vi "Correlation_Display.vi"(5 "Inst names":string[](array[string])=["HW 1", "HW 2"], 6 "OK":bool) -> (2 "correlation array":i32[][](array[numeric]) min=0 max=8)   [LabVIEW 2010]
uses:
  Globals/Meas_global.vi
panel:
  in  "number of correlation pairs":i32=1
  in  "correlation choices":i32[][](array[ring])=[[0, 1], [0, 0], [0, 0]] items=["LDA (U)", "LDA (W)", "HW (HW) Sync", "RV (WT) Sync", "HW (HW)", "RV (WT)"]
  # "1st Pair"
  # "2nd Pair"
  # "3rd Pair"
  # "4th Pair"
  # "5th Pair"
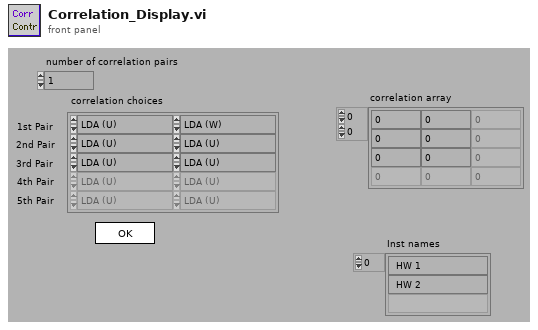
[diagram p1: front panel]
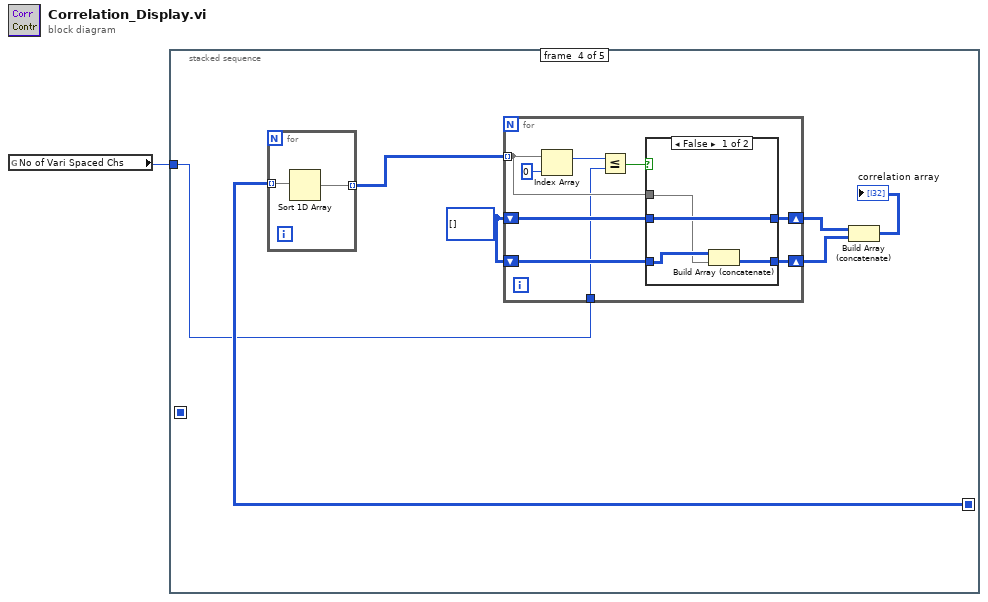
[diagram p0: block diagram]
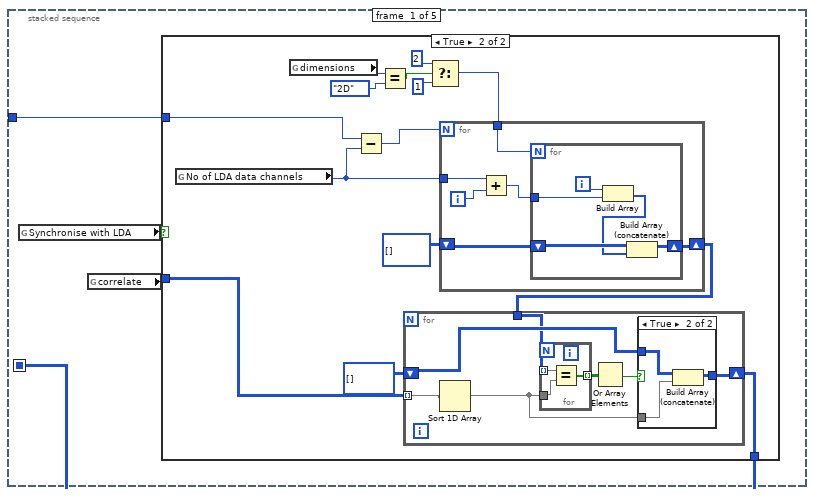
[diagram p2: hidden frame]
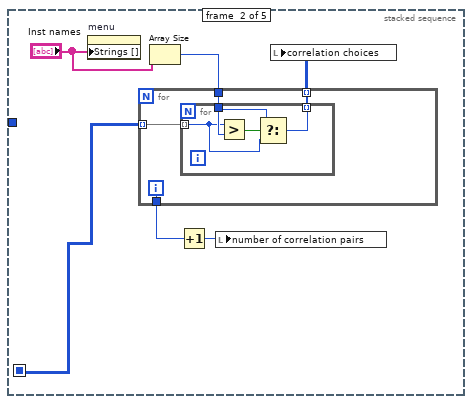
[diagram p5: hidden frame]
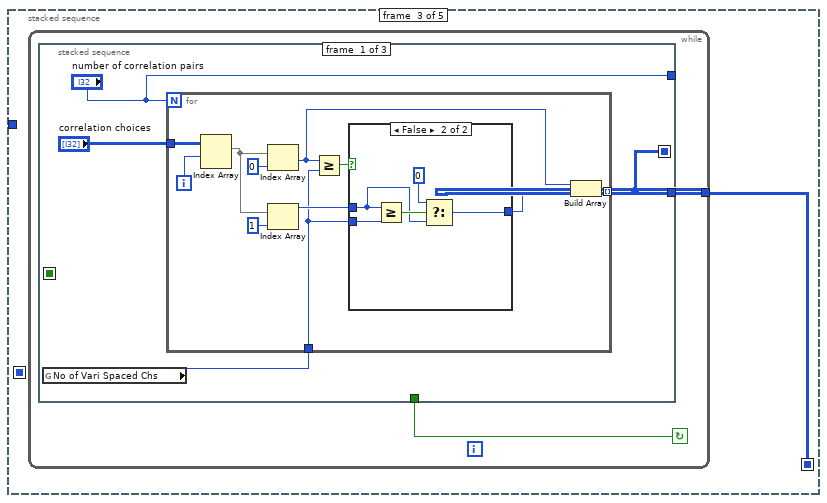
[diagram p6: hidden frame]
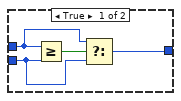
[diagram p7: hidden frame]
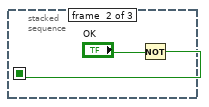
[diagram p8: hidden frame]
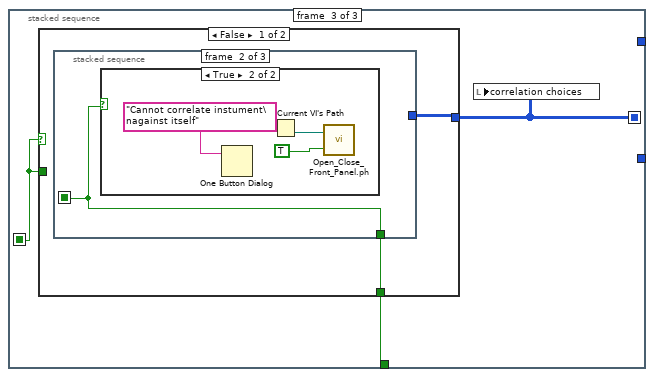
[diagram p9: hidden frame]
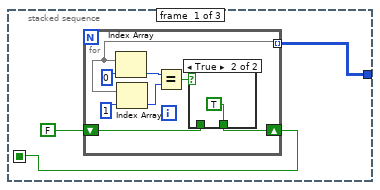
[diagram p10: hidden frame]
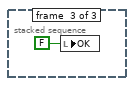
[diagram p13: hidden frame]
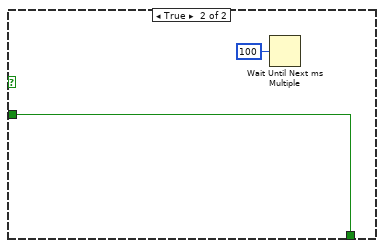
[diagram p14: hidden frame]
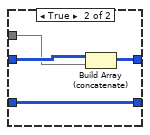
[diagram p15: hidden frame]
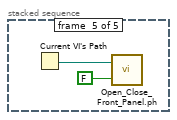
[diagram p16: hidden frame]
diagram:
  n1 = global read "Meas_global.vi" "No of Vari Spaced Chs"() -> (w1:i32)
  n2 = stacked-sequence {
    seq-local: [_ _ w60 _ _] -> [_ _ _ w120 _]
    seq-local: [w3 _ _ _ _] -> [_ w48 _ _ _]
    tunnel: w1 -> [w2 _ _ w117 _]
    frame #0 {
      n3 = global read "Meas_global.vi" "Synchronise with LDA"() -> (w5:bool)
      n4 = global read "Meas_global.vi" "correlate"() -> (w4:i32[][])
      n5 = case shown="True" w5 {
        tunnel: w4 -> [w6 w12]
        tunnel: [w6 w11] -> w3
        tunnel: w2 -> [_ w9]
        frame False {
        }
        frame True {
          n6 = global read "Meas_global.vi" "No of LDA data channels"() -> (w19:i32)
          n7 = global read "Meas_global.vi" "dimensions"() -> (w18:enum16{"1D", "2D"})
          n8 = Subtract(x=w9, y=w19) -> (x-y=w20:i32)
          n9 = Equal?(x=w18, y=enum16{"1D", "2D"}."2D" ("dimensions")) -> (x = y?=w16:bool)
          n10 = Select(t=2, s=w16, f=1) -> (s? t:f=w13:i32)
          n11 = for {
            N: w20 -> [_]
            tunnel: w19 -> [w40]
            tunnel: w13 -> [w38]
            shift-right: [w36] -> w7
            shift-left: i32[][] [] -> [w35]
            i -> [w39]
            n12 = Add(x=w40, y=w39) -> (x+y=w37:i32)
            n13 = for {
              N: w38 -> [_]
              tunnel: w37 -> [w44]
              shift-right: [w42] -> w36
              shift-left: w35 -> [w43]
              i -> [w45]
              n14 = Build Array(w45, w44) -> (w41:i32[])
              n15 = Build Array (concatenate)(w43, w41) -> (w42:i32[][])
            }
          }
          n16 = for {
            shift-right: [w25] -> w11
            shift-left: i32[][] [] -> [w22]
            tunnel: w12 -> [w24] mode=indexing
            tunnel: w7 -> [w21]
            n17 = Sort 1D Array(array=w24) -> (sorted array=w23:i32[])
            n18 = for {
              tunnel: w23 -> [w34]
              tunnel: w21 -> [w32] mode=indexing
              tunnel: [w33] -> w27 mode=indexing
              tunnel: w21 -> [_] mode=indexing
              n19 = Equal?(x=w32, y=w34) -> (x = y?=w33:bool[])
            }
            n20 = Or Array Elements(Boolean array=w27) -> (logical OR=w26:bool)
            n21 = case shown="True" w26 {
              tunnel: [w28 w30] -> w25
              tunnel: w22 -> [w28 w31]
              tunnel: w23 -> [_ w29]
              frame False {
              }
              frame True {
                n22 = Build Array (concatenate)(w31, w29) -> (w30:i32[][])
              }
            }
          }
        }
      }
    }
    frame #1 {
      n23 = property on="menu" class="Ring (strict)"("Strings []"="Inst names") -> ()  [unwired: 2 in, 2 out]
      n24 = Array Size(array="Inst names") -> (size(s)=w49:i32)
      n25 = for {
        tunnel: w49 -> [w55]
        tunnel: w48 -> [w54] mode=indexing
        tunnel: [w53] -> w50 mode=indexing
        tunnel: [w52] -> w47
        i -> [w52]
        n26 = for {
          tunnel: w55 -> [w58]
          tunnel: w54 -> [w57] mode=indexing
          tunnel: [w56] -> w53 mode=indexing
          n27 = Greater?(x=w57, y=w58) -> (0:w59:bool)
          n28 = Select(t=w58, s=w59, f=w57) -> (s? t:f=w56:i32)
        }
      }
      n29 = Increment(x=w47) -> (x+1=w46:i32)
      n30 = local write "number of correlation pairs"(w46) -> ()
      n31 = local write "correlation choices"(w50) -> ()
    }
    frame #2 {
      n32 = while {
        tunnel: [w62] -> w60
        stop <- w61 continue-if-true
        n33 = stacked-sequence {
          seq-local: [w64 _ _] -> [_ _ w89]
          seq-local: [_ w88 _] -> [_ _ w90]
          tunnel: [w64 _ _] -> w62
          tunnel: [_ _ w91] -> w61
          tunnel: ["number of correlation pairs" _ _] -> _
          frame #0 {
            n34 = global read "Meas_global.vi" "No of Vari Spaced Chs"() -> (w63:i32)
            n35 = for {
              N: "number of correlation pairs" -> [_]
              tunnel: "correlation choices" -> [w76]
              tunnel: w63 -> [w69]
              tunnel: [w71] -> w64 mode=indexing
              i -> [w77]
              n36 = Index Array(array=w76, index (row)=w77) -> (element=w73:i32[])  [unwired: 1 in]
              n37 = Index Array(array=w73, index=0 ("Index")) -> (element=w67:i32)
              n38 = Index Array(array=w73, index=1 ("Index")) -> (element=w70:i32)
              n39 = Greater Or Equal?(x=w67, y=w69) -> (x >= y?=w72:bool)
              n40 = case shown="False" w72 {
                tunnel: w70 -> [w80 w83]
                tunnel: w69 -> [w78 w84]
                tunnel: [w79 w85] -> w68
                frame True {
                  n41 = Greater Or Equal?(x=w80, y=w78) -> (x >= y?=w81:bool)
                  n42 = Select(t=w80, s=w81, f=w78) -> (s? t:f=w79:i32)
                }
                frame False {
                  n43 = Greater Or Equal?(x=w83, y=w84) -> (x >= y?=w86:bool)
                  n44 = Select(t=i8 0, s=w86, f=w83) -> (s? t:f=w85:i32)
                }
              }
              n45 = Build Array(w67, w68) -> (w71:i32[])
            }
          }
          frame #1 {
            n46 = Not(x="OK") -> (.not. x?=w88:bool)
          }
          frame #2 {
            n47 = case shown="False" w90 {
              tunnel: w89 -> [w93 _]
              tunnel: [w92 w113] -> w91
              tunnel: w90 -> [_ w113]
              frame False {
                n48 = stacked-sequence {
                  seq-local: [w94 _ _] -> [_ w107 _]
                  tunnel: w93 -> [w96 _ _]
                  tunnel: [_ w107 _] -> w92
                  frame #0 {
                    n49 = for {
                      tunnel: w96 -> [w100] mode=indexing
                      shift-right: [w98] -> w94
                      shift-left: FALSE -> [w97]
                      n50 = Index Array(array=w100, index=0) -> (element=w102:i32)
                      n51 = Index Array(array=w100, index=1) -> (element=w101:i32)
                      n52 = Equal?(x=w102, y=w101) -> (x = y?=w99:bool)
                      n53 = case shown="True" w99 {
                        tunnel: [w105 TRUE] -> w98
                        tunnel: w97 -> [w105 _]
                        frame False {
                        }
                        frame True {
                        }
                      }
                    }
                  }
                  frame #1 {
                    n54 = case shown="True" w107 {
                      frame False {
                      }
                      frame True {
                        n55 = One Button Dialog(message="Cannot correlate instument\nagainst itself") -> ()  [unwired: 2 out]
                        n56 = Current VI's Path() -> (path=w109:path)
                        n57 = call "Open_Close_Front_Panel.ph.vi"("Front Panel Window:Open"=TRUE, "VI path"=w109) -> ()  [unwired: 2 out]
                      }
                    }
                  }
                  frame #2 {
                    n58 = local write "OK"(FALSE ("OK")) -> ()
                  }
                }
              }
              frame True {
                n59 = Wait Until Next ms Multiple(millisecond multiple=u32 100) -> ()  [unwired: 1 out]
              }
            }
            n60 = local write "correlation choices"(w89) -> ()
          }
        }
      }
    }
    frame #3 {
      w119 = i32[][] []
      n61 = for {
        tunnel: w120 -> [w139] mode=indexing
        tunnel: [w138] -> w118 mode=indexing
        n62 = Sort 1D Array(array=w139) -> (sorted array=w138:i32[])
      }
      n63 = for {
        tunnel: w118 -> [w125] mode=indexing
        tunnel: w117 -> [w121]
        shift-right: [w124] -> w115
        shift-left: w119 -> [w126]
        shift-right: [w122] -> w116
        shift-left: w119 -> [w123]
        n64 = Index Array(array=w125, index=0 ("Index")) -> (element=w128:i32)
        n65 = Less Or Equal?(x=w128, y=w121) -> (x <= y?=w127:bool)
        n66 = case shown="False" w127 {
          tunnel: w126 -> [w131 w137]
          tunnel: w125 -> [w130 w136]
          tunnel: [w131 w135] -> w124
          tunnel: w123 -> [w133 w134]
          tunnel: [w132 w134] -> w122
          frame False {
            n67 = Build Array (concatenate)(w133, w130) -> (w132:i32[][])
          }
          frame True {
            n68 = Build Array (concatenate)(w137, w136) -> (w135:i32[][])
          }
        }
      }
      n69 = Build Array (concatenate)(w115, w116) -> (→"correlation array":i32[][])
    }
    frame #4 {
      n70 = Current VI's Path() -> (path=w141:path)
      n71 = call "Open_Close_Front_Panel.ph.vi"("Front Panel Window:Open"=FALSE, "VI path"=w141) -> ()  [unwired: 2 out]
    }
  }
